vi "Event_enemy_passiveness.vi"(8 "error in (no error)":errorcluster, 10 "EnemyRobots":refnum<class "Robot.lvclass">[](array[class]), 11 "Events in":refnum<class "Events.lvclass">) -> (0 "error out":errorcluster, 3 "Events out":refnum<class "Events.lvclass">)   [LabVIEW 2023, in "Events.lvclass"]
uses:
  Events.lvclass
  Robot_class/Robot.lvclass
  C:/Users/ebert/Documents/codes/SSL/repo/SSL_AI/Object_class/Object.lvclass
  Object_class/Object.lvclass/Object.ctl
  Object_class/Read x.vi
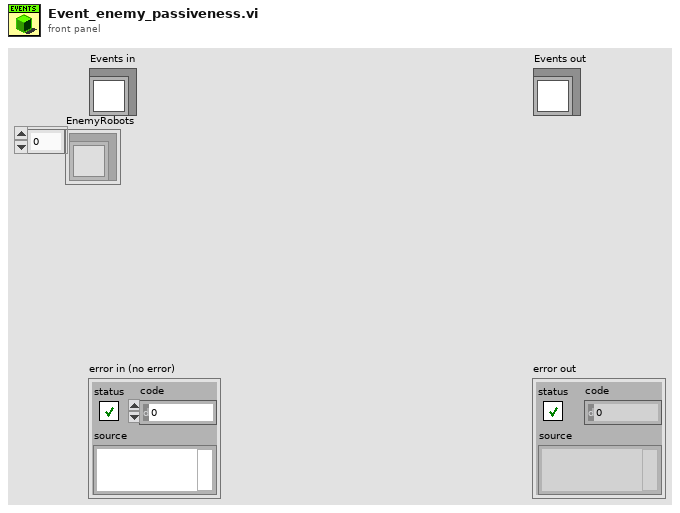
[diagram p1: front panel]
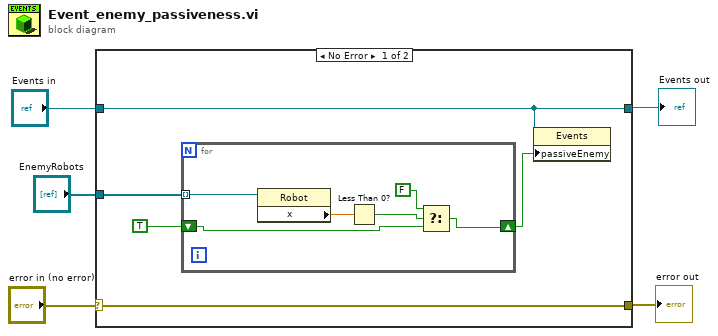
[diagram p0: block diagram]
diagram:
  n1 = case shown="No Error" "error in (no error)" {
    selector: "error in (no error)" -> [w10 w18]
    tunnel: [w10 w18] -> w4
    tunnel: [w9 w17] -> w2
    tunnel: "Events in" -> [w9 w17]
    tunnel: "EnemyRobots" -> [w7 _]
    frame No Error {
      n2 = for {
        shift-right: [w11] -> w6
        shift-left: TRUE -> [w12]
        tunnel: w7 -> [w16] mode=indexing
        n3 = property class="Robot"(reference=w16) -> ("x"=w15:dbl)  [unwired: 1 in, 2 out]
        n4 = Less Than 0?(x=w15) -> (x < 0?=w14:bool)
        n5 = Select(t=FALSE, s=w14, f=w12) -> (s? t:f=w11:bool)
      }
      n6 = property class="Events"(reference=w9, "passiveEnemy"=w6) -> ()  [unwired: 1 in, 2 out]
    }
    frame Error {
    }
  }
  "error out" <- w4
  "Events out" <- w2
